vi "JSON to LVObject.vi"(8 "error in (no error)":errorcluster, 9 "JSON":string, 10 "Offset of first non-whitespace":i32, 11 "LabVIEW Object in":refnum<class>) -> (0 "error out":errorcluster, 3 "LabVIEW Object out":refnum<class>)   [LabVIEW 2024, in "JSONtext.lvlib"]
uses:
  JSONtext.lvlib
  Advance past String.vi
  String Subset.vi
  Strip Quotes and Unescape.vi
  Unescape JSON string.vi
  Parsing Error in converting to LabVIEW type.vi
  Base64 Support.lvlib
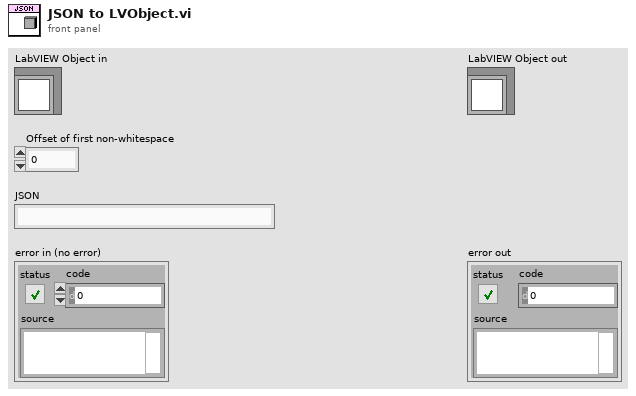
[diagram p1: front panel]
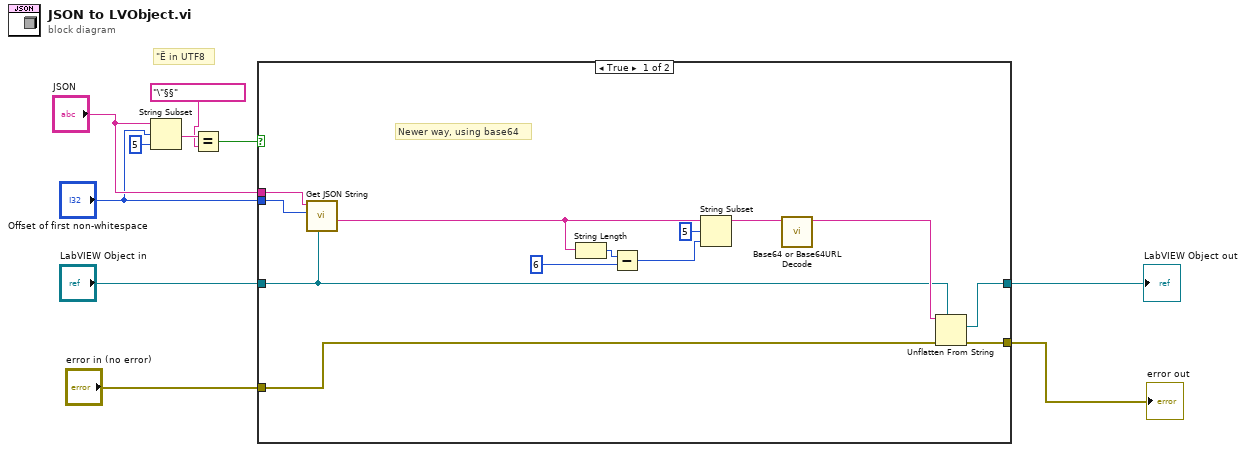
[diagram p0: block diagram]
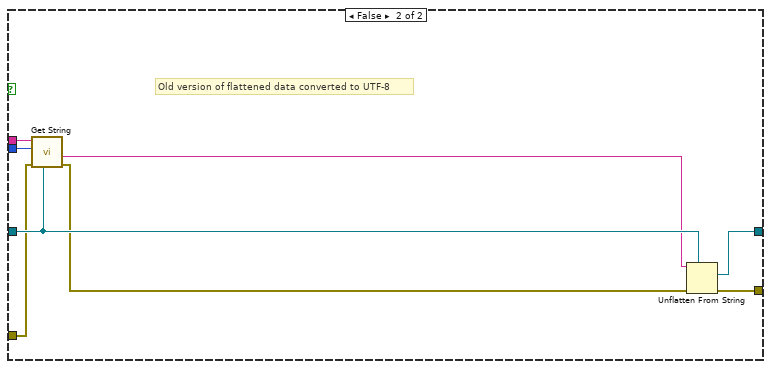
[diagram p2: hidden frame]
diagram:
  # "\"Ё in UTF8"
  n1 = String Subset(string="JSON", offset (0)="Offset of first non-whitespace", length (rest)=5 ("length (rest)")) -> (substring=w4:string)
  n2 = Equal?(x=w4, y="\"§§" ("string")) -> (x = y?=w2:bool)
  n3 = case shown="True" w2 {
    tunnel: "LabVIEW Object in" -> [w11 w31]
    tunnel: [w23 w30] -> w9
    tunnel: [w22 w29] -> w8
    tunnel: "Offset of first non-whitespace" -> [w14 w28]
    tunnel: "error in (no error)" -> [w18 w26]
    tunnel: "JSON" -> [w13 w24]
    frame True {
      # "Newer way, using base64"
      n4 = call "Get JSON String.vi"("LV Type"=w11, "Offset"=w14, "JSON"=w13) -> ("<JSON>String"=w12:string)  [unwired: 6 in, 2 out]
      n5 = String Length(string=w12) -> (length=w17:i32)
      n6 = Subtract(x=w17, y=6) -> (x-y=w15:i32)
      n7 = String Subset(string=w12, offset (0)=5, length (rest)=w15) -> (substring=w20:string)
      n8 = call "Base64 or Base64URL Decode.vi"("Base64 or Base64URL"=w20) -> ("Decoded"=w21:string)  [unwired: 10 in]
      n9 = Unflatten From String(type=w11, binary string=w21, error in (no error)=w18) -> (value=w22:refnum<class>, error out=w23:errorcluster)  [unwired: 2 in, 1 out]
    }
    frame False {
      # "Old version of flattened data converted to UTF-8"
      n10 = call "Get String.vi"("LV Type"=w31, "error in (no error)"=w26, "Offset"=w28, "JSON"=w24) -> ("error out"=w25:errorcluster, "String"=w27:string)  [unwired: 5 in, 1 out]
      n11 = Unflatten From String(type=w31, binary string=w27, error in (no error)=w25) -> (value=w29:refnum<class>, error out=w30:errorcluster)  [unwired: 2 in, 1 out]
    }
  }
  "error out" <- w9
  "LabVIEW Object out" <- w8
